vi "Controls on Panel.vi"(8 "error in (no error)":errorcluster, 11 "VI Refnum in":refnum<vi>) -> (0 "error out":errorcluster, 2 "ControlOnPanel":refnum<vi>[](array[refnum]), 3 "VI Refnum out":refnum<vi>)   [LabVIEW 2017, in "Toolbox.lvlib"]
uses:
  Toolbox.lvlib
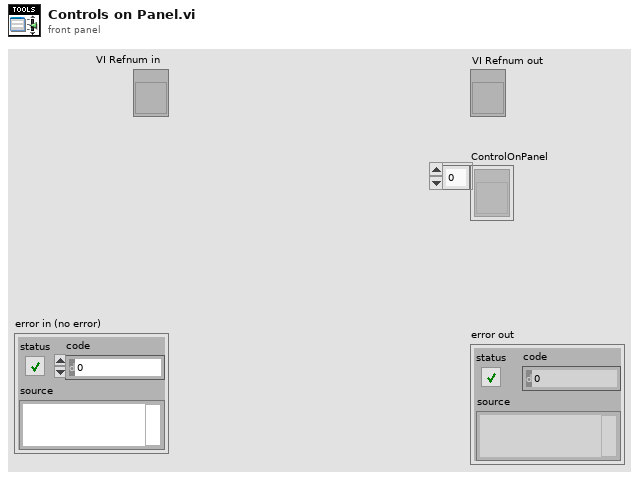
[diagram p1: front panel]
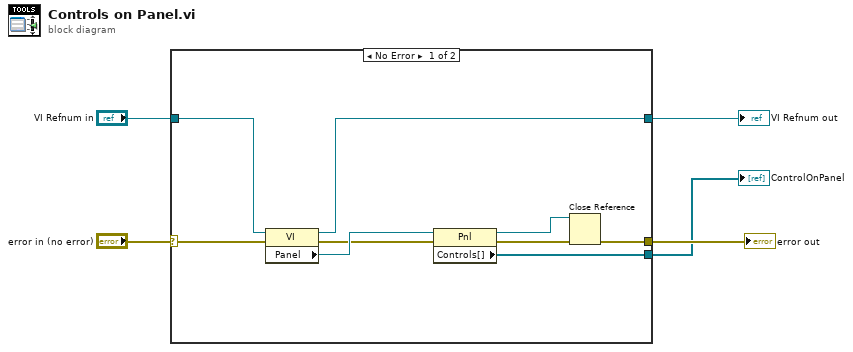
[diagram p0: block diagram]
diagram:
  n1 = case shown="No Error" "error in (no error)" {
    selector: "error in (no error)" -> [w14 w16]
    tunnel: [w8 w16] -> w4
    tunnel: "VI Refnum in" -> [w13 w15]
    tunnel: [w9 w15] -> w2
    tunnel: [w6 _] -> w1
    frame No Error {
      n2 = property class="VI"(reference=w13, error in=w14) -> (reference out=w9:refnum<vi>, error out=w11:errorcluster, "Panel"=w12:refnum<vi>)
      n3 = property class="Pnl"(reference=w12, error in=w11) -> (reference out=w7:refnum<vi>, error out=w10:errorcluster, "Controls[]"=w6:refnum<vi>[])
      n4 = Close Reference(reference=w7, error in (no error)=w10) -> (error out=w8:errorcluster)
    }
    frame Error {
    }
  }
  "error out" <- w4
  "VI Refnum out" <- w2
  "ControlOnPanel" <- w1
